vi "Frame Data Increment.vi"(7 "Len":u8, 11 "Data in":u8[](array[numeric])) -> (3 "Data out":u8[](array[numeric]))   [LabVIEW 2011, in "CAN FD.lvlib"]
uses:
  CAN FD.lvlib
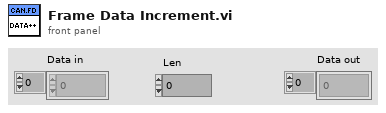
[diagram p1: front panel]
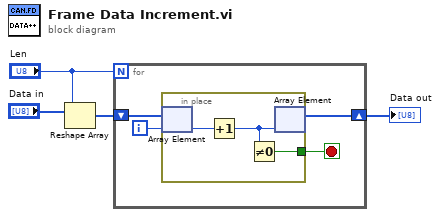
[diagram p0: block diagram]
diagram:
  n1 = Reshape Array("Data in", "Len") -> (w3:u8[])
  n2 = for {
    N: "Len" -> [_]
    shift-right: [w6] -> w1
    shift-left: w3 -> [w8]
    i -> [w7]
    stop <- w5 stop-if-true
    n3 = in-place {
      in-place-border: [w9] -> w5
      n4 = in-place-array #1(w8, w7) -> (w11:u8)
      n5 = Increment(x=w11) -> (x+1=w10:u8)
      n6 = Not Equal To 0?(x=w10) -> (x != 0?=w9:bool)
      n7 = in-place-array #1(w10) -> (w6:u8[])  [unwired: 1 out]
    }
  }
  "Data out" <- w1
